vi "Motion_Wait for Load.vi"(8 "error in":errorcluster, 9 "poll interval (0.1s)":dbl[unit]=0.1, 10 "timeout (10s)":dbl[unit]=10.0 caption="Time Target (s)" format="%.1f", 11 "TCP refnum":refnum<k5>) -> (0 "error out":errorcluster, 1 "Loader At Load":bool, 2 "Loader At Connect":bool, 3 "TCP refnum dup":refnum<k5>, 4 "timeout error":bool, 5 "elapsed time":dbl[unit]=nan format="%.1f", 6 "done":bool)   [LabVIEW 2010]
doc: "This function polls the Motion Control Loader discretes until the Loader is at a terminal position, a time-out occurs, or an error occurs. A Stopwatch popup displays the elapsed time while polling occurs."
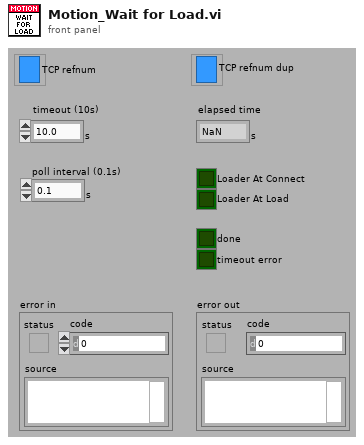
[diagram p1: front panel]
types:
  T1 = cluster{"Loader Enabled":bool, "Loader Alarm ":bool, "Loader Warning":bool, "Loader At Connect":bool, "Loader At Load":bool, "Loader Connect Aborted":bool, "Loader Connect Error":bool, "Loader Connecting":bool, "Loader Control Alarm":bool, "Loader At Home":bool, "Loader Home Error":bool, "Loader Home Aborted":bool, "Loader Homing":bool, "Loader Load Aborted":bool, "Loader Load Error":bool, "Loader Loading":bool, "Loader Stop Aborted":bool, "Loader Stop Error":bool, "Loader Stopped":bool, "Loader Stopping":bool, "Loader General Alarm":bool, "Motion Alarm":bool, "Loader Home Required":bool}
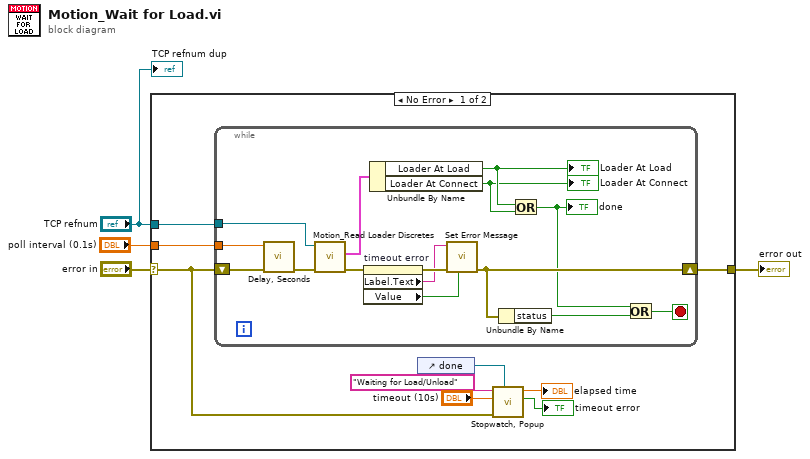
[diagram p0: block diagram]
diagram:
  n1 = case shown="No Error" "error in" {
    selector: "error in" -> [w6 w29]
    tunnel: "TCP refnum" -> [w8 _]
    tunnel: [w7 w29] -> w4
    tunnel: "poll interval (0.1s)" -> [w5 _]
    frame No Error {
      n2 = while {
        tunnel: w8 -> [w28]
        shift-right: [w20] -> w7
        shift-left: w6 -> [w26]
        tunnel: w5 -> [w14]
        stop <- w17 stop-if-true
        n3 = call "Delay, Seconds.vi"("error in"=w26, "delay"=w14) -> ("error out"=w25:errorcluster)  [unwired: 5 in, 1 out]
        n4 = call "Motion_Read Loader Discretes.vi"("error in (no error)"=w25, "TCP Connection Refnum in"=w28) -> ("error out"=w24:errorcluster, "Loader Discretes"=w27:T1)  [unwired: 7 in, 1 out]
        n5 = property on="timeout error" class="Bool (strict)"(error in=w24) -> (error out=w23:errorcluster, "Label.Text"=w21:string, "Value"=w22:bool)  [unwired: 1 in, 1 out]
        n6 = Unbundle By Name(w27) -> ("Loader At Load"=w19:bool, "Loader At Connect"=w18:bool)
        "Loader At Load" <- w19
        "Loader At Connect" <- w18
        n7 = call "Set Error Message.vi"("enable (T)"=w22, "error in"=w23, "message"=w21) -> ("error out"=w20:errorcluster)  [unwired: 5 in]
        n8 = Unbundle By Name(w20) -> ("status"=w16:bool)
        n9 = Or(x=w19, y=w18) -> (x .or. y?=w15:bool)
        "done" <- w15
        n10 = Or(x=w15, y=w16) -> (x .or. y?=w17:bool)
      }
      n11 = control-ref of="done"() -> (w12:refnum<vi>)
      n12 = call "Stopwatch, Popup.vi"("Stop (Bool) Refnum"=w12, "error in (no error)"=w6, "Time Target"="timeout (10s)", "Front Panel Window:Title"="Waiting for Load/Unload") -> ("Time has Elapsed"=→"timeout error":bool, "Elapsed Time (Knob)"=→"elapsed time":dbl[unit])  [unwired: 5 in, 1 out]
    }
    frame Error {
    }
  }
  "error out" <- w4
  "TCP refnum dup" <- "TCP refnum"
